vi "subHamamatsu_CloseCam.vi"(7 "Live":bool, 8 "error in (no error)":errorcluster, 11 "Handle in":u32) -> (0 "error out":errorcluster)   [LabVIEW 2015]
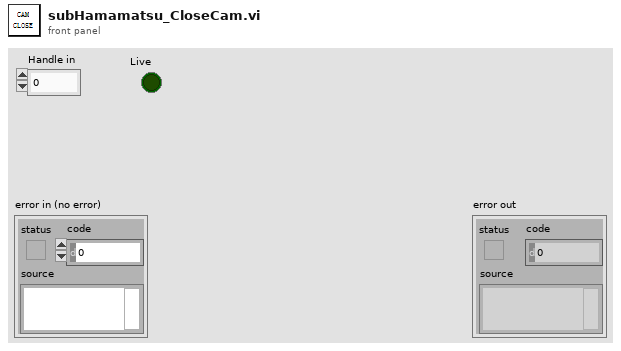
[diagram p1: front panel]
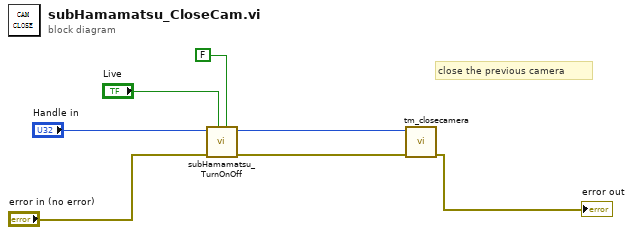
[diagram p0: block diagram]
diagram:
  # "close the previous camera"
  n1 = call "subHamamatsu_TurnOnOff.vi"("logic 2"=FALSE ("Start/Stop Capture"), "logic 1"="Live", "error in (no error)"="error in (no error)", "Handle in"="Handle in") -> ("error out"=w7:errorcluster, "Handle out"=w2:u32)  [unwired: 5 in, 1 out]
  n2 = call "tm_closecamera.vi"("error in (no error)"=w7, "Handle in"=w2) -> ("error out"=→"error out":errorcluster)  [unwired: 9 in]
